vi "Init User List.vi"(8 "error in (no error)":errorcluster, 11 "[V] Login in":refnum<class "[V] Login.lvclass">) -> (0 "error out":errorcluster, 3 "[V] Login out":refnum<class "[V] Login.lvclass">)   [LabVIEW 2020, in "[V] Login.lvlib" / "[V] Login.lvclass"]
uses:
  [V] Login.lvclass
  [V] Login.lvclass/[V] Login.ctl
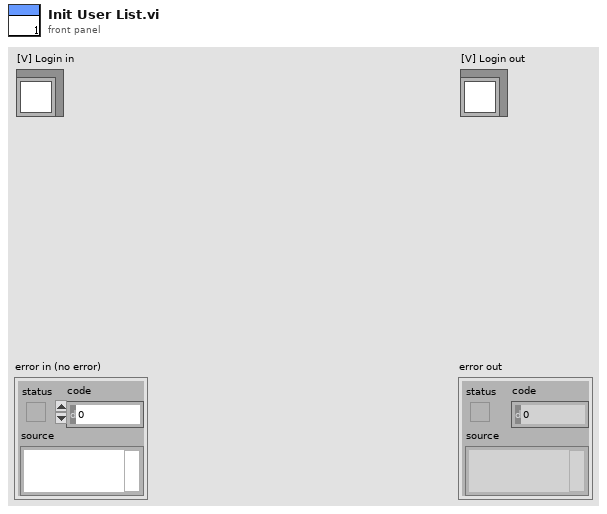
[diagram p1: front panel]
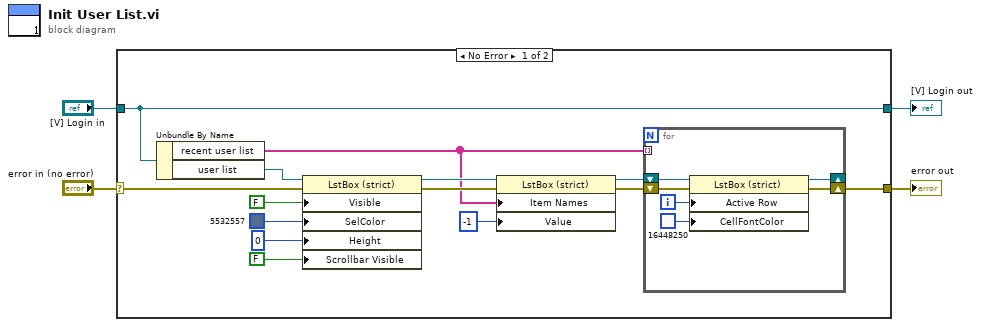
[diagram p0: block diagram]
diagram:
  n1 = case shown="No Error" "error in (no error)" {
    selector: "error in (no error)" -> [w17 w26]
    tunnel: [w6 w26] -> w3
    tunnel: [w18 w25] -> w1
    tunnel: "[V] Login in" -> [w18 w25]
    frame No Error {
      n2 = Unbundle By Name(w18) -> ("recent user list"=w5:string[], "user list"=w16:refnum<vi>)
      n3 = property class="LstBox (strict)"(reference=w16, error in=w17, "Visible"=FALSE, "SelColor"=u32 5532557 ("Selection Color"), "Height"=u32 0 ("Size:Height"), "Scrollbar Visible"=FALSE ("Visible Items:Vertical Scrollbar Visible")) -> (reference out=w13:refnum<vi>, error out=w14:errorcluster)
      n4 = property class="LstBox (strict)"(reference=w13, error in=w14, "Item Names"=w5, "Value"=-1) -> (reference out=w8:refnum<vi>, error out=w7:errorcluster)
      n5 = for {
        shift-right: [w19] -> _
        shift-left: w8 -> [w23]
        shift-right: [w20] -> w6
        shift-left: w7 -> [w24]
        tunnel: w5 -> [_] mode=indexing
        i -> [w22]
        n6 = property class="LstBox (strict)"(reference=w23, error in=w24, "Active Row"=w22, "CellFontColor"=u32 16448250 ("Selection Color")) -> (reference out=w19:refnum<vi>, error out=w20:errorcluster)
      }
    }
    frame Error {
    }
  }
  "error out" <- w3
  "[V] Login out" <- w1
